vi "AddPoints.vi"(10 "Old List":dbl[][](array[numeric]), 11 "New List":dbl[][](array[numeric])) -> (1 "Y":u32[](array[numeric]), 2 "X":u32[](array[numeric]))   [LabVIEW 2017, in "AODControl.lvlib"]
uses:
  AODControl.lvlib
  CodifyFrequency(Array).vi
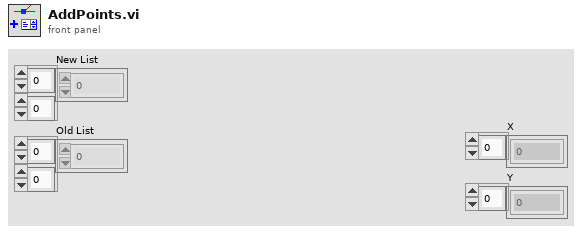
[diagram p1: front panel]
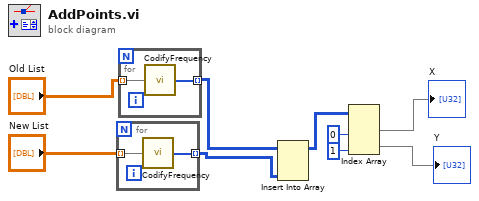
[diagram p0: block diagram]
diagram:
  n1 = for {
    tunnel: "New List" -> [w11] mode=indexing
    tunnel: [w10] -> w2 mode=indexing
    n2 = call-poly "CodifyFrequency.vi"("Array"=w11) -> ("Array 2"=w10:u32[])
  }
  n3 = for {
    tunnel: "Old List" -> [w13] mode=indexing
    tunnel: [w12] -> w3 mode=indexing
    n4 = call-poly "CodifyFrequency.vi"("Array"=w13) -> ("Array 2"=w12:u32[])
  }
  n5 = Insert Into Array(array=w3, new element=w2) -> (w1:u32[][])  [unwired: 2 in]
  n6 = Index Array(array=w1, index (col) #1=0 ("disabled index (col)"), index (col) #2=1 ("index (col)")) -> (element #1=→"X":u32[], element #2=→"Y":u32[])  [unwired: 2 in]
